vi "Helper - Overlay waypoints.vi"(9 "Shape to Overlay":bool[][](array[boolean])=[[TRUE, TRUE, TRUE, TRUE, TRUE, TRUE, TRUE, FALSE, FALSE, FALSE, TRUE, TRUE, TRUE, TRUE, TRUE, TRUE, TRUE, FALSE], [TRUE, TRUE, TRUE, TRUE, TRUE, TRUE, FALSE, FALSE, FALSE, FALSE, FALSE, TRUE, TRUE, TRUE, TRUE, TRUE, TRUE, FALSE], [TRUE, TRUE, TRUE, TRUE, TRUE, FALSE, FALSE, TRUE, TRUE, TRUE, FALSE, FALSE, TRUE, TRUE, TRUE, TRUE, TRUE, FALSE], [TRUE, TRUE, TRUE, TRUE, FALSE, FALSE, FALSE, TRUE, TRUE, TRUE, FALSE, FALSE, FALSE, TRUE, TRUE, TRUE, TRUE, FALSE], [TRUE, TRUE, TRUE, FALSE, FALSE, FALSE, FALSE, TRUE, TRUE, TRUE, FALSE, FALSE, FALSE, FALSE, TRUE, TRUE, TRUE, FALSE], [TRUE, TRUE, FALSE, FALSE, FALSE, FALSE, FALSE, TRUE, TRUE, TRUE, FALSE, FALSE, FALSE, FALSE, FALSE, TRUE, TRUE, FALSE], [TRUE, FALSE, FALSE, FALSE, FALSE, FALSE, FALSE, TRUE, TRUE, TRUE, FALSE, FALSE, FALSE, FALSE, FALSE, FALSE, TRUE, FALSE], [FALSE, FALSE, TRUE, TRUE, TRUE, TRUE, TRUE, TRUE, TRUE, TRUE, TRUE, TRUE, TRUE, TRUE, TRUE, FALSE, FALSE, FALSE], [FALSE, FALSE, TRUE, TRUE, TRUE, TRUE, TRUE, TRUE, TRUE, TRUE, TRUE, TRUE, TRUE, TRUE, TRUE, FALSE, FALSE, FALSE], [FALSE, FALSE, TRUE, TRUE, TRUE, TRUE, TRUE, TRUE, TRUE, TRUE, TRUE, TRUE, TRUE, TRUE, TRUE, FALSE, FALSE, FALSE], [TRUE, FALSE, FALSE, FALSE, FALSE, FALSE, FALSE, TRUE, TRUE, TRUE, FALSE, FALSE, FALSE, FALSE, FALSE, FALSE, TRUE, FALSE], [TRUE, TRUE, FALSE, FALSE, FALSE, FALSE, FALSE, TRUE, TRUE, TRUE, FALSE, FALSE, FALSE, FALSE, FALSE, TRUE, TRUE, FALSE], [TRUE, TRUE, TRUE, FALSE, FALSE, FALSE, FALSE, TRUE, TRUE, TRUE, FALSE, FALSE, FALSE, FALSE, TRUE, TRUE, TRUE, FALSE], [TRUE, TRUE, TRUE, TRUE, FALSE, FALSE, FALSE, TRUE, TRUE, TRUE, FALSE, FALSE, FALSE, TRUE, TRUE, TRUE, TRUE, FALSE], [TRUE, TRUE, TRUE, TRUE, TRUE, FALSE, FALSE, TRUE, TRUE, TRUE, FALSE, FALSE, TRUE, TRUE, TRUE, TRUE, TRUE, FALSE], [TRUE, TRUE, TRUE, TRUE, TRUE, TRUE, FALSE, FALSE, FALSE, FALSE, FALSE, TRUE, TRUE, TRUE, TRUE, TRUE, TRUE, FALSE], [TRUE, TRUE, TRUE, TRUE, TRUE, TRUE, TRUE, FALSE, FALSE, FALSE, TRUE, TRUE, TRUE, TRUE, TRUE, TRUE, TRUE, FALSE]], 10 "Color to Overlay":u32(colorbox)=16711680, 11 "Img Refnum in":T1) -> (3 "Img Refnum out":T1)   [LabVIEW 2011]
doc: "Given an image, reads the current list of waypoints off of the global variable and overlays their UTM-to-pixel conversions on the image.\n\nPurpose: Allows us to see our waypoints on an overview map or overhead camera image.\n\nAuthor: Jason Curtis"
uses:
  <vilib>/vision/Image Controls.llb/IMAQ Image.ctl
  2 Globals/2 Global.vi
panel:
  in  "Image Descriptor Path":path=path "../../1,3 C-Small RC Platform/LPB Pool Image Descriptor.txt"
  out "overlayed locations":cluster{"X":i32, "Y":i32}[](array[cluster])
  out "Bitmap to overlay":u32[][](array[colorbox])
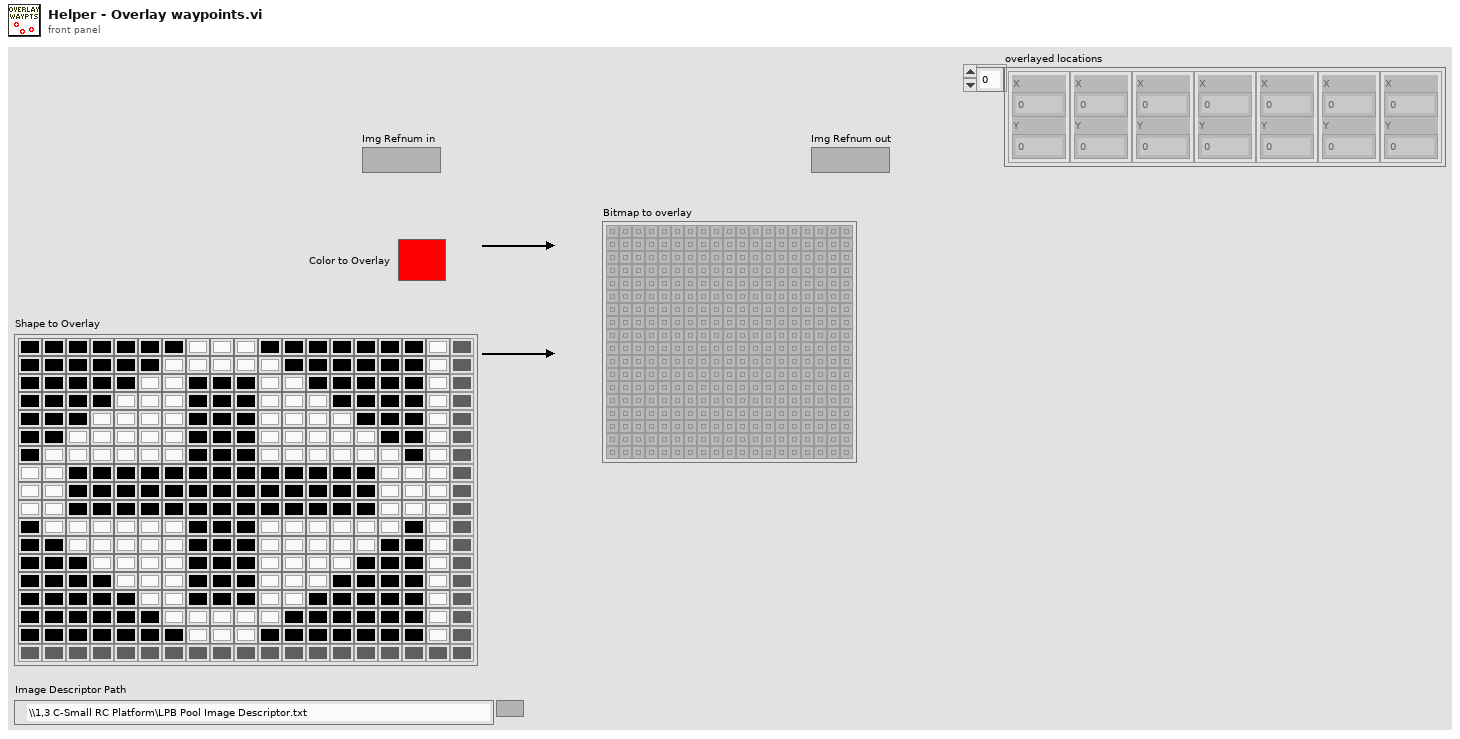
[diagram p1: front panel]
types:
  T1 = typedef "IMAQ Image.ctl" = refnum<image>
  T2 = typedef "0-Image Descriptor.ctl" = cluster{"Upper-Left Corner Coordinates":T3, "Meters/Pixel":dbl}
  T3 = typedef "UTM Location.ctl" = cluster{"UTM Zone":dbl, "Hemisphere":enum16{"North", "South"}, "East":dbl, "North":dbl}
  T4 = typedef "Waypoints List.ctl" = T5[]
  T5 = typedef "ocuWaypoint.ctl" = cluster{"Point Type":T6, "Dist/Time":dbl, "UTM Location":T3}
  T6 = typedef "waypointTypes.ctl" = enum16{"Drive", "Round Port", "Round Starboard", "Stay"}
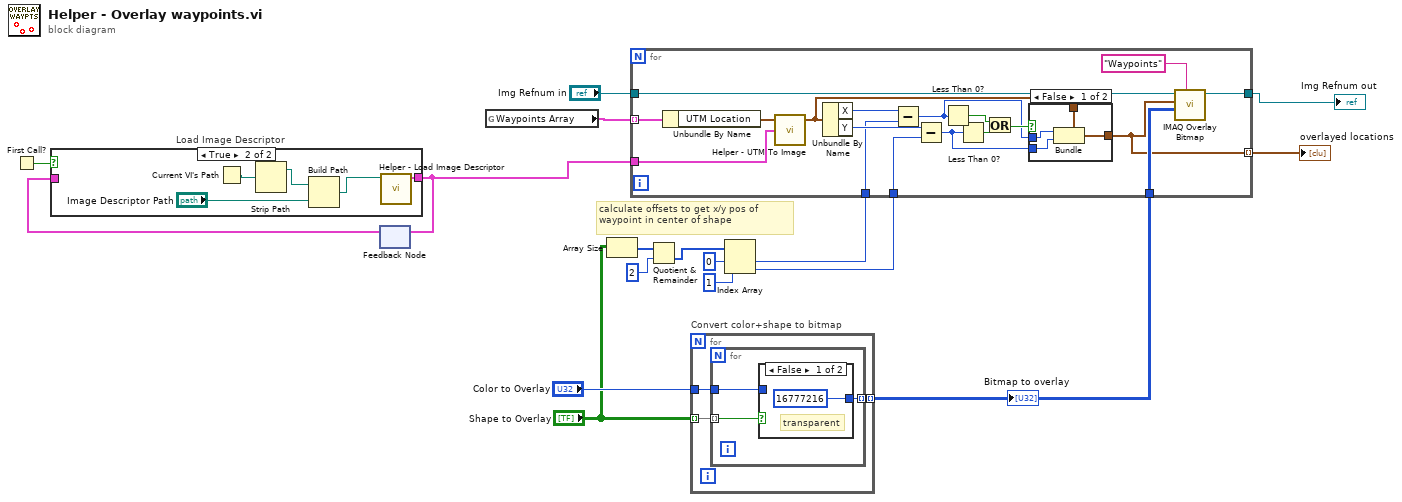
[diagram p0: block diagram]
diagram:
  # "calculate offsets to get x/y pos of waypoint in center of shape"
  n1 = First Call?() -> (First Call?: T/F=w3:bool)
  n2 = feedback #1() -> (w1:T2)  [unwired: 1 in]
  n3 = case "Load Image Descriptor" shown="True" w3 {
    tunnel: [w18 w23] -> w2
    tunnel: w1 -> [w18 _]
    frame False {
    }
    frame True {
      n4 = Current VI's Path() -> (path=w21:path)
      n5 = Strip Path(path=w21) -> (stripped path=w20:path)  [unwired: 1 out]
      n6 = Build Path(base path=w20, name or relative path="Image Descriptor Path") -> (appended path=w19:path)
      n7 = call "Helper - Load Image Descriptor.vi"("Image Descriptor File Path"=w19) -> ("Image Descriptor Typedef out"=w23:T2)  [unwired: 10 in]
    }
  }
  n8 = feedback-in #1(w2) -> ()
  n9 = global read "2 Global.vi" "Waypoints Array"() -> (w4:T4)
  n10 = Array Size(array="Shape to Overlay") -> (size(s)=w9:i32[])
  n11 = Quotient & Remainder(x=w9, y=2 ("index")) -> (floor(x/y)=w7:i32[])  [unwired: 1 out]
  n12 = for "Convert color+shape to bitmap" {
    tunnel: "Shape to Overlay" -> [w26] mode=indexing
    tunnel: [w25] -> w14 mode=indexing
    tunnel: "Color to Overlay" -> [w24]
    n13 = for {
      tunnel: w26 -> [w29] mode=indexing
      tunnel: [w28] -> w25 mode=indexing
      tunnel: w24 -> [w27]
      n14 = case shown="False" w29 {
        tunnel: [u32 16777216 ("element") w31] -> w28
        tunnel: w27 -> [_ w31]
        frame False {
          # "transparent"
        }
        frame True {
        }
      }
    }
  }
  "Bitmap to overlay" <- w14
  n15 = Index Array(array=w7, index #1=0 ("index"), index #2=1 ("index")) -> (element #1=w6:i32, element #2=w10:i32)
  n16 = for {
    tunnel: "Img Refnum in" -> [w47]
    tunnel: [w48] -> w16
    tunnel: w4 -> [w49] mode=indexing
    tunnel: w14 -> [w45]
    tunnel: w6 -> [w43]
    tunnel: w10 -> [w42]
    tunnel: [w35] -> w5 mode=indexing
    tunnel: w2 -> [w34]
    n17 = Unbundle By Name(w49) -> ("UTM Location"=w33:T3)
    n18 = call "Helper - UTM To Image.vi"("Image Descriptor"=w34, "UTM Location"=w33) -> ("Pixel Coordinates"=w32:cluster{"X":i32, "Y":i32})  [unwired: 1 in, 2 out]
    n19 = Unbundle By Name(w32) -> ("X"=w41:i32, "Y"=w44:i32)
    n20 = Subtract(x=w41, y=w43) -> (x-y=w37:i32)
    n21 = Subtract(x=w44, y=w42) -> (x-y=w36:i32)
    n22 = Less Than 0?(x=w37) -> (x < 0?=w40:bool)
    n23 = Less Than 0?(x=w36) -> (x < 0?=w39:bool)
    n24 = Or(x=w40, y=w39) -> (x .or. y?=w38:bool)
    n25 = case shown="False" w38 {
      tunnel: w32 -> [w53 w54]
      tunnel: w37 -> [w52 _]
      tunnel: w36 -> [w51 _]
      tunnel: [w50 w54] -> w35
      frame False {
        n26 = Bundle(cluster=w53, "X"=w52, "Y"=w51) -> (w50:cluster{"X":i32, "Y":i32})
      }
      frame True {
      }
    }
    n27 = call "IMAQ Overlay Bitmap"("Group"="Waypoints", "Bitmap"=w45, "Top Left Point"=w35, "Image"=w47) -> ("Image Out"=w48:T1)  [unwired: 6 in, 1 out]
  }
  "Img Refnum out" <- w16
  "overlayed locations" <- w5
